vi "Control Panel Speed Control.vi"() -> (2 "Turn":dbl=-0.0, 3 "Speed":dbl)   [LabVIEW 2019]
uses:
  Framework/Robot Global Data.vi
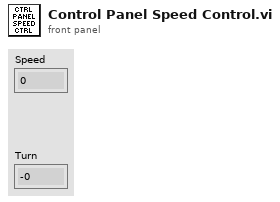
[diagram p1: front panel]
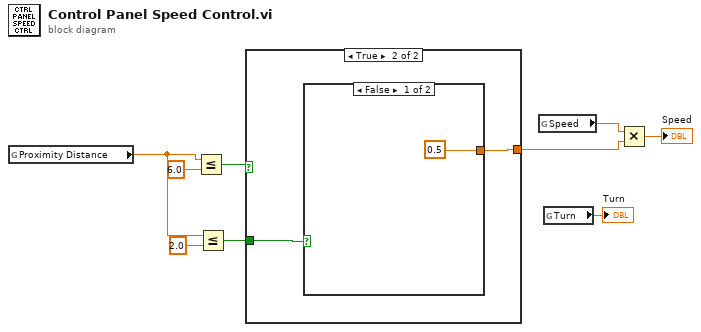
[diagram p0: block diagram]
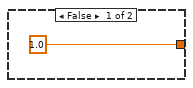
[diagram p2: hidden frame]
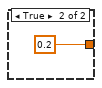
[diagram p3: hidden frame]
diagram:
  n1 = global read "Robot Global Data.vi" "Proximity Distance"() -> (w8:dbl)
  n2 = Less Or Equal?(x=w8, y=6.0) -> (x <= y?=w5:bool)
  n3 = Less Or Equal?(x=w8, y=2.0) -> (x <= y?=w3:bool)
  n4 = case shown="True" w5 {
    tunnel: [1.0 ("f") w11] -> w4
    tunnel: w3 -> [_ w12]
    frame False {
    }
    frame True {
      n5 = case shown="False" w12 {
        tunnel: [0.5 ("t") 0.2 ("t")] -> w11
        frame False {
        }
        frame True {
        }
      }
    }
  }
  n6 = global read "Robot Global Data.vi" "Speed"() -> (w6:dbl)
  n7 = global read "Robot Global Data.vi" "Turn"() -> (→"Turn":dbl)
  n8 = Multiply(x=w6, y=w4) -> (x*y=→"Speed":dbl)
